vi "Util_Trajectory_WriteFile_OneState.vi"(9 "TRAJ_STATE":T1={"TimeSeconds"=0.0, "Velocity"=0.0, "Acceleration"=0.0, "POSE"={"TRANSLATION"={"X"=0.0, "Y"=0.0}, "ROTATION"={"VALUE"=0.0, "COS"=1.0, "SIN"=0.0}}, "Curvature"=0.0} {"POSE"."ROTATION"."SIN" format="%13.4f"; "POSE"."ROTATION"."COS" format="%13.4f"; "POSE"."ROTATION"."VALUE" format="%13.4f"; "POSE"."TRANSLATION"."Y" format="%14.3f"; "POSE"."TRANSLATION"."X" format="%14.3f"}, 10 "Comment":string, 11 "Byte Stream File in":refnum<file>) -> (3 "Byte Stream File out":refnum<file>)   [LabVIEW 2019, in "Trajectory_Library.lvlib"]
doc: "Internal subVI used by Util_Trajectory_WriteFile (and others). This writes one trajectory state to a file.\n\nParameters:\n - Byte stream in - file stream\n - comment - comment for this line\n - TrajectoryState - The state to write\n\nReturns: \n - Byte Stream Out - file stream"
uses:
  Trajectory_Library.lvlib
  TypeDef/TRAJ_STATE.ctl
  TypeDef/POSE2D.ctl
  TypeDef/TRANSLATION2D.ctl
  TypeDef/ROTATION2D.ctl
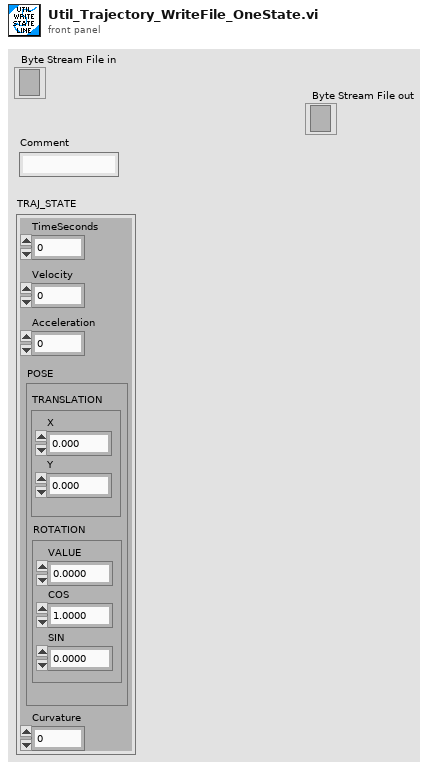
[diagram p1: front panel]
types:
  T1 = typedef "Trajectory_Library.lvlib/TRAJ_STATE.ctl" = cluster{"TimeSeconds":dbl, "Velocity":dbl, "Acceleration":dbl, "POSE":T2, "Curvature":dbl}
  T2 = typedef "Trajectory_Library.lvlib/POSE2D.ctl" = cluster{"TRANSLATION":T3, "ROTATION":T4}
  T3 = typedef "Trajectory_Library.lvlib/TRANSLATION2D.ctl" = cluster{"X":dbl, "Y":dbl}
  T4 = typedef "Trajectory_Library.lvlib/ROTATION2D.ctl" = cluster{"VALUE":dbl, "COS":dbl, "SIN":dbl}
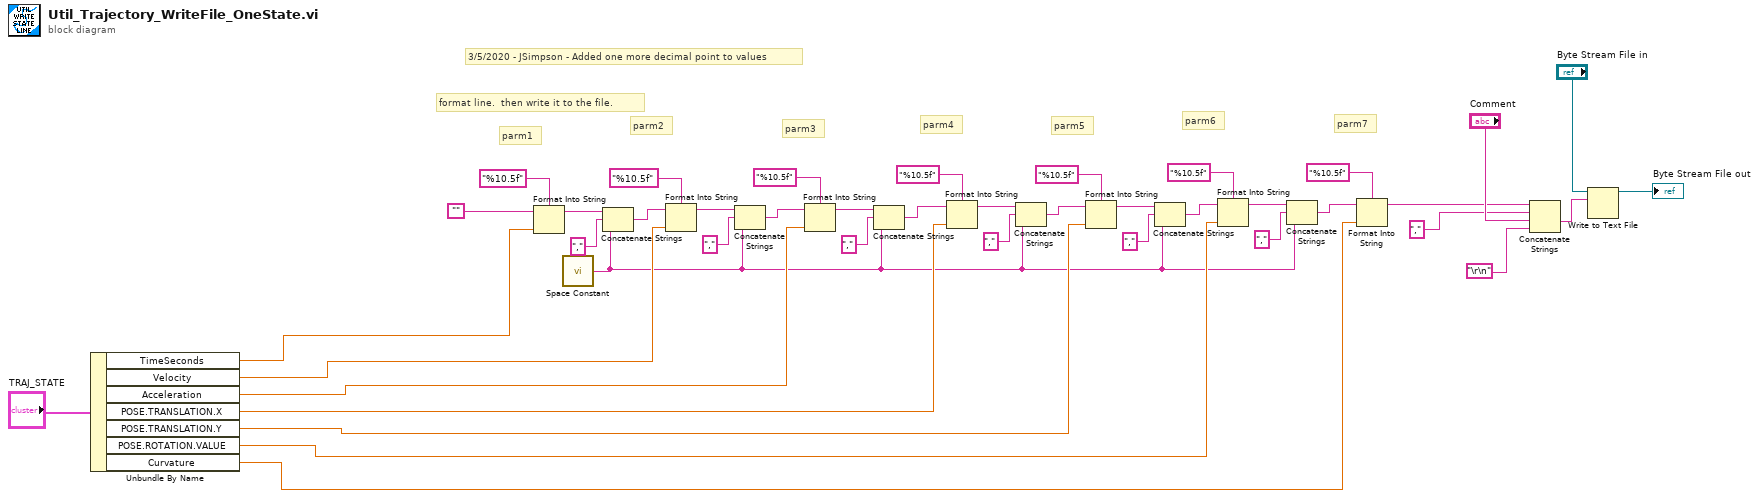
[diagram p0: block diagram]
diagram:
  # "3/5/2020 - JSimpson - Added one more decimal point to values"
  # "format line.  then write it to the file."
  # "parm7"
  # "parm6"
  # "parm5"
  # "parm4"
  # "parm3"
  # "parm2"
  # "parm1"
  n1 = Unbundle By Name("TRAJ_STATE") -> ("TimeSeconds"=w9:dbl, "Velocity"=w8:dbl, "Acceleration"=w7:dbl, "POSE.TRANSLATION.X"=w6:dbl, "POSE.TRANSLATION.Y"=w5:dbl, "POSE.ROTATION.VALUE"=w4:dbl, "Curvature"=w3:dbl)
  n2 = Format Into String(format string="%10.5f", initial string="", w9) -> (resulting string=w13:string)  [unwired: 1 in, 1 out]
  n3 = call <vilib>:"Space Constant.vi"() -> ("String"=w1:string)
  n4 = Concatenate Strings(w13, "," ("string"), w1) -> (w23:string)
  n5 = Format Into String(format string="%10.5f", initial string=w23, w8) -> (resulting string=w16:string)  [unwired: 1 in, 1 out]
  n6 = Concatenate Strings(w16, "," ("string"), w1) -> (w22:string)
  n7 = Format Into String(format string="%10.5f", initial string=w22, w7) -> (resulting string=w19:string)  [unwired: 1 in, 1 out]
  n8 = Concatenate Strings(w19, "," ("string"), w1) -> (w37:string)
  n9 = Format Into String(format string="%10.5f", initial string=w37, w6) -> (resulting string=w24:string)  [unwired: 1 in, 1 out]
  n10 = Concatenate Strings(w24, "," ("string"), w1) -> (w30:string)
  n11 = Format Into String(format string="%10.5f", initial string=w30, w5) -> (resulting string=w27:string)  [unwired: 1 in, 1 out]
  n12 = Concatenate Strings(w27, "," ("string"), w1) -> (w36:string)
  n13 = Format Into String(format string="%10.5f", initial string=w36, w4) -> (resulting string=w31:string)  [unwired: 1 in, 1 out]
  n14 = Concatenate Strings(w31, "," ("string"), w1) -> (w35:string)
  n15 = Format Into String(format string="%10.5f", initial string=w35, w3) -> (resulting string=w2:string)  [unwired: 1 in, 1 out]
  n16 = Concatenate Strings(w2, "," ("string"), "Comment", "\r\n") -> (w39:string)
  n17 = Write to Text File(file (use dialog)="Byte Stream File in", text=w39) -> (refnum out=→"Byte Stream File out":refnum<file>)  [unwired: 2 in, 2 out]
